vi "determineNewLogFilePath.vi"(8 "error in (no error)":errorcluster, 11 "Logger in":refnum<class "Log.lvclass">) -> (0 "error out":errorcluster, 2 "logFilePath":path, 3 "Logger out":refnum<class "Log.lvclass">)   [LabVIEW 2013, in "Log.lvlib" / "Log.lvclass"]
uses:
  <userlib>/Common/Log/Log/Log.lvclass
  <userlib>/Common/Log/Log/Log.lvclass/Log.ctl
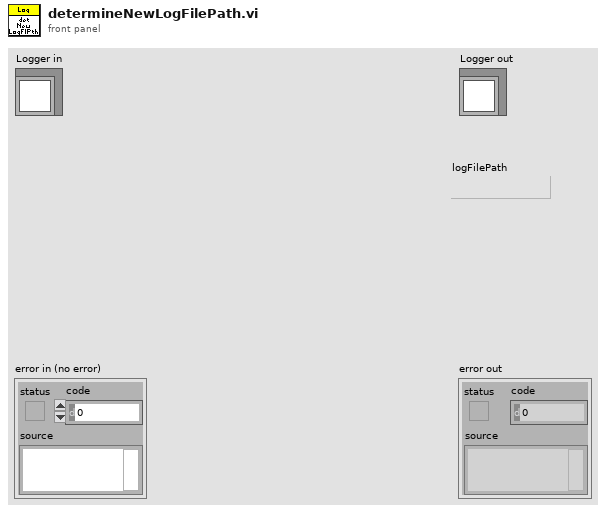
[diagram p1: front panel]
types:
  T1 = enum16{"open", "replace", "create", "open or create", "replace or create", "replace or create with confirmation"}
  T2 = enum16{"open", "open or create", "create or replace", "create", "open (read-only)"}
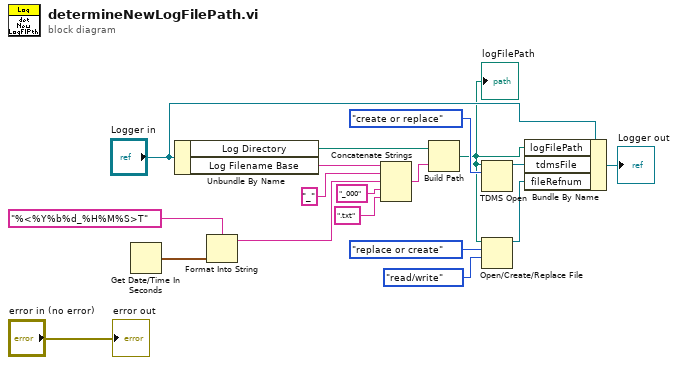
[diagram p0: block diagram]
diagram:
  n1 = Get Date/Time In Seconds() -> (seconds since 1Jan1904=w13:timestamp)
  n2 = Unbundle By Name("Logger in") -> ("Log Directory"=w9:path, "Log Filename Base"=w7:string)
  n3 = Format Into String(format string="%<%Y%b%d_%H%M%S>T", w13) -> (resulting string=w16:string)  [unwired: 2 in, 1 out]
  n4 = Concatenate Strings(w7, "_" ("string"), w16, "_000" ("string"), ".txt" ("string")) -> (w14:string)
  n5 = Build Path(base path=w9, name or relative path=w14) -> (appended path=w4:path)
  "logFilePath" <- w4
  n6 = TDMS Open(10:T2."create or replace" ("operation (0:open)"), 11:w4) -> (3:w5:refnum<k34>)  [unwired: 5 in, 1 out]
  n7 = Open/Create/Replace File(file path (use dialog)=w4, operation (0:open)=T1."replace or create", access (0:read/write)=enum16{"read/write", "read-only", "write-only"}."read/write") -> (refnum out=w1:refnum<file>)  [unwired: 3 in, 2 out]
  n8 = Bundle By Name(cluster="Logger in", "logFilePath"=w4, "tdmsFile"=w5, "fileRefnum"=w1) -> (→"Logger out":refnum<class "Log.lvclass">)
  "error out" <- "error in (no error)"
